vi "Up Down Counter FGV.vi"(7 "操作选择":T1=enum."加1", 8 "错误输入":cluster{"状态":bool, "代码":i32, "源":string}) -> (0 "错误输出":cluster{"状态":bool, "代码":i32, "源":string}, 2 "运行总数":i32)   [LabVIEW 2012]
uses:
  Up Down Counter Command.ctl
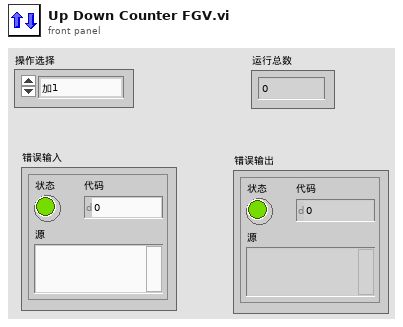
[diagram p1: front panel]
types:
  T1 = typedef "Up Down Counter Command.ctl" = enum16{"重置", "加1", "减1", "获取当前值"}
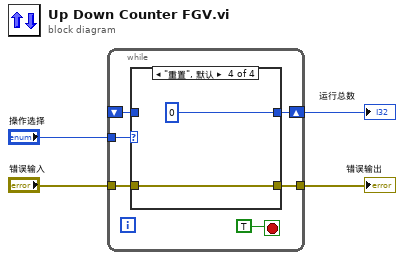
[diagram p0: block diagram]
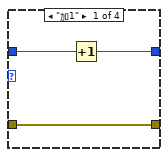
[diagram p2: hidden frame]
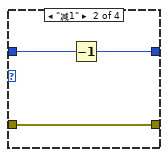
[diagram p3: hidden frame]
diagram:
  n1 = while {
    tunnel: "操作选择" -> [w9]
    tunnel: "错误输入" -> [w8]
    tunnel: [w7] -> w2
    shift-right: [w6] -> w1
    shift-left: _ -> [w5]
    stop <- TRUE stop-if-true
    n2 = case shown="\"重置\", 默认" w9 {
      tunnel: w8 -> [w13 w16 w18 w20]
      tunnel: [w13 w16 w18 w20] -> w7
      tunnel: [w11 w14 w17 0] -> w6
      tunnel: w5 -> [w12 w15 w17 _]
      frame "加1" {
        n3 = Increment ("加1")(x=w12) -> (x+1=w11:i32)
      }
      frame "减1" {
        n4 = Decrement ("减1")(x=w15) -> (x-1=w14:i32)
      }
      frame "获取当前值" {
      }
      frame "重置", Default {
      }
    }
  }
  "运行总数" <- w1
  "错误输出" <- w2
